vi "change tag select data type.vi"(7 "data type":T1, 8 "error in":errorcluster, 10 "tag select name":string, 11 "tag select  module configuration in":refnum<class "tag select module configuration.lvclass">) -> (0 "error out":errorcluster, 2 "changed channels":refnum<class "TBM channel.lvclass">[](array[class]), 3 "tag select module configuration out":refnum<class "tag select module configuration.lvclass">)   [LabVIEW 2015, in "tag select module configuration.lvclass"]
uses:
  tag select module configuration.lvclass
  <vilib>/NI/Tag Bus/tag/Data Type.ctl
  <vilib>/NI/Tag Bus Module Framework/channel/TBM channel.lvclass
  <vilib>/NI/Tag Bus/tag/tag descriptor.lvclass/tag descriptor.ctl
  tag select module configuration.lvclass/tag select module configuration.ctl
  <vilib>/NI/Tag Bus/tag/tag descriptor.lvclass
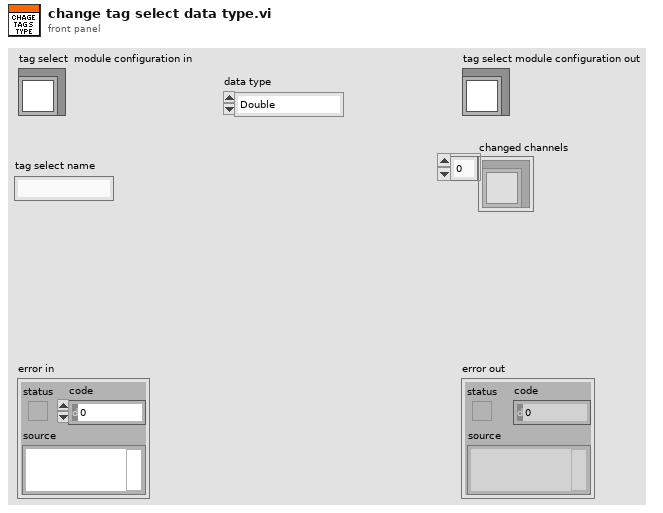
[diagram p1: front panel]
types:
  T1 = typedef "tag bus.lvlib/tag descriptor.lvclass/Data Type.ctl" = enum16{"Double", "Single", "I64", "I32", "I16", "I8", "U64", "U32", "U16", "U8", "Boolean", "String", "Array of Double", "Array of Single", "Array of I64", "Array of I32", "Array of I16", "Array of I8", "Array of U64", "Array of U32", "Array of U16", "Array of U8", "Array of Boolean", "Array of String"}
  T2 = typedef "tag select module configuration.lvclass/tag select configuration.ctl" = cluster{"tag select name":string, "data type":T1, "output":refnum<class "TBM channel.lvclass">, "select":refnum<class "TBM channel.lvclass">, "input channels":refnum<class "TBM channel.lvclass">[]}
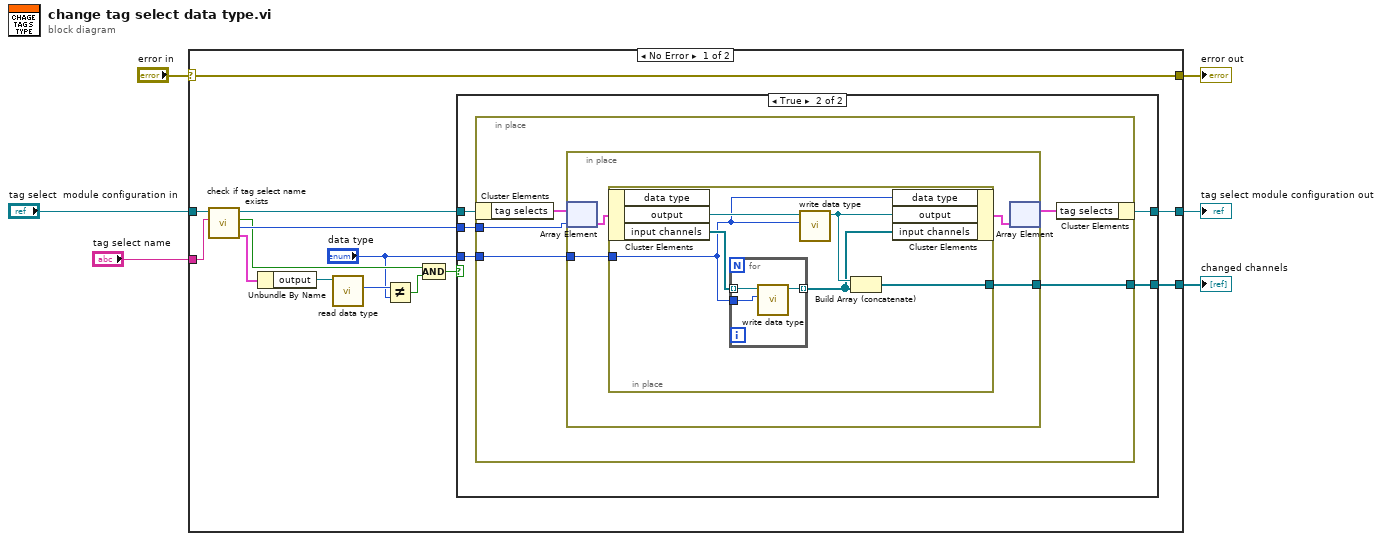
[diagram p0: block diagram]
diagram:
  n1 = case shown="No Error" "error in" {
    selector: "error in" -> [w7 w46]
    tunnel: "tag select  module configuration in" -> [w20 w45]
    tunnel: "tag select name" -> [w19 _]
    tunnel: [w10 _] -> w4
    tunnel: [w9 w45] -> w3
    tunnel: [w7 w46] -> w1
    frame No Error {
      n2 = call "check if tag select name exists.vi"("name to locate"=w19, "tag select module configuration in"=w20) -> ("tag select config"=w16:T2, "index"=w17:i32, "found?"=w13:bool, "tag select module configuration out"=w18:refnum<class "tag select module configuration.lvclass">)  [unwired: 6 in]
      n3 = Unbundle By Name(w16) -> ("output"=w15:refnum<class "TBM channel.lvclass">)
      n4 = call <vilib>:"read data type.vi"("system tag in"=w15) -> ("data type"=w14:T1)  [unwired: 8 in, 2 out]
      n5 = Not Equal?(x=w14, y="data type") -> (x != y?=w12:bool)
      n6 = Compound Arithmetic op=AND(w13, w12) -> (w11:bool)
      n7 = case shown="True" w11 {
        tunnel: w18 -> [w21 w26]
        tunnel: [w21 w25] -> w9
        tunnel: w17 -> [_ w24]
        tunnel: [_ w23] -> w10
        tunnel: "data type" -> [_ w22]
        frame False {
        }
        frame True {
          n8 = in-place {
            in-place-border: w24 -> [w29]
            in-place-border: [w28] -> w23
            in-place-border: w22 -> [w27]
            n9 = in-place-cluster #1(w26) -> ("tag selects"=w31:T2[])
            n10 = in-place {
              in-place-border: [w33] -> w28
              in-place-border: w27 -> [w32]
              n11 = in-place-array #2(w31, w29) -> (w35:T2)
              n12 = in-place {
                in-place-border: [w40] -> w33
                in-place-border: w32 -> [w36]
                n13 = in-place-cluster #3(w35) -> ("output"=w39:refnum<class "TBM channel.lvclass">, "input channels"=w41:refnum<class "TBM channel.lvclass">[])  [unwired: 1 out]
                n14 = for {
                  tunnel: w41 -> [w43] mode=indexing
                  tunnel: [w44] -> w37 mode=indexing
                  tunnel: w36 -> [w42]
                  n15 = call <vilib>:"write data type.vi"("data type"=w42, "system tag in"=w43) -> ("system tag out"=w44:refnum<class "TBM channel.lvclass">)  [unwired: 8 in, 1 out]
                }
                n16 = call <vilib>:"write data type.vi"("data type"=w36, "system tag in"=w39) -> ("system tag out"=w38:refnum<class "TBM channel.lvclass">)  [unwired: 8 in, 1 out]
                n17 = Build Array (concatenate)(w38, w37) -> (w40:refnum<class "TBM channel.lvclass">[])
                n18 = in-place-cluster #3("data type"=w36, "output"=w38, "input channels"=w37) -> (w34:T2)
              }
              n19 = in-place-array #2(w34) -> (w30:T2[])  [unwired: 1 out]
            }
            n20 = in-place-cluster #1("tag selects"=w30) -> (w25:refnum<class "tag select module configuration.lvclass">)
          }
        }
      }
    }
    frame Error {
    }
  }
  "error out" <- w1
  "tag select module configuration out" <- w3
  "changed channels" <- w4
